vi "Subvi probe DIO31 D0.vi"(9 "D0":bool) -> ()   [LabVIEW 2017]
uses:
  <vilib>/rvi/eio/common/nirviEmuTemplateMethod_errors.vi
  <vilib>/eio/EIONode/EIONode.xnode
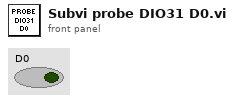
[diagram p1: front panel]
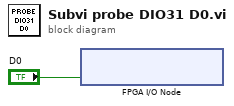
[diagram p0: block diagram]
diagram:
  n1 = xnode "FPGA I/O Node"("Connector0/DIO31"="D0") -> ()  [unwired: 1 in, 1 out]
